vi "Delete Diagram SubVIs.vi"(8 "error in (no error)":errorcluster, 11 "Diagram in":refnum<vi>) -> (0 "error out":errorcluster, 3 "Diagram out":refnum<vi>)   [LabVIEW 2019, in "gRPC Template Creation Utility.lvlib"]
uses:
  gRPC Template Creation Utility.lvlib
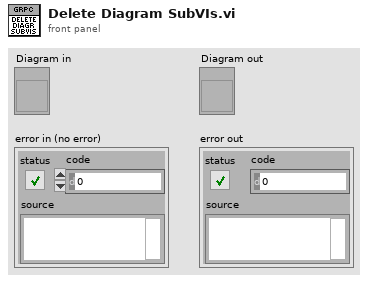
[diagram p1: front panel]
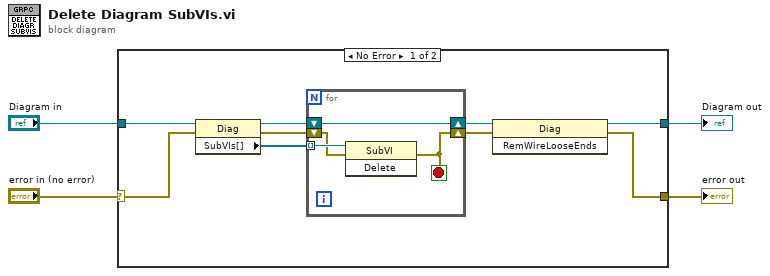
[diagram p0: block diagram]
diagram:
  n1 = case shown="No Error" "error in (no error)" {
    selector: "error in (no error)" -> [w9 w18]
    tunnel: [w6 w19] -> w4
    tunnel: [w5 w18] -> w3
    tunnel: "Diagram in" -> [w10 w19]
    frame No Error {
      n2 = property class="Diag"(reference=w10, error in=w9) -> (reference out=w13:refnum<vi>, error out=w12:errorcluster, "SubVIs[]"=w11:refnum<vi>[])
      n3 = for {
        tunnel: w11 -> [w17] mode=indexing
        shift-right: [w14] -> w7
        shift-left: w12 -> [w15]
        shift-right: [w16] -> w8
        shift-left: w13 -> [w16]
        stop <- w14 stop-if-true
        n4 = invoke class="SubVI" method="Delete"(reference=w17, error in=w15) -> (error out=w14:errorcluster)  [unwired: 1 in, 2 out]
      }
      n5 = invoke class="Diag" method="RemWireLooseEnds"(reference=w8, error in=w7) -> (reference out=w6:refnum<vi>, error out=w5:errorcluster)  [unwired: 1 in, 1 out]
    }
    frame Error {
    }
  }
  "Diagram out" <- w4
  "error out" <- w3
